vi "determineConfigTabUIPath.vi"(8 "error in (no error)":errorcluster, 11 "ConfigurationTabUI in":refnum<class "ConfigurationTabUI.lvclass">) -> (0 "error out":errorcluster, 2 "cfgTabUIPath":path, 3 "ConfigurationTabUI out":refnum<class "ConfigurationTabUI.lvclass">)   [LabVIEW 2012, in "ExampleConfiguration.lvlib" / "ConfigurationTabUI.lvclass"]
doc: "Determines the path to configTabUI.vi."
uses:
  ConfigurationTabUI.lvclass
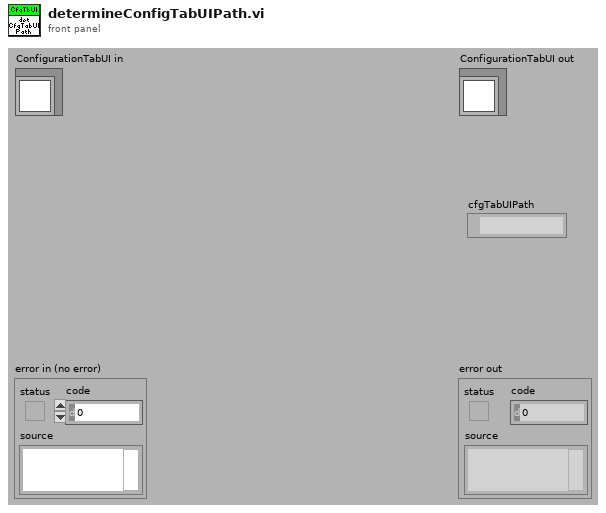
[diagram p1: front panel]
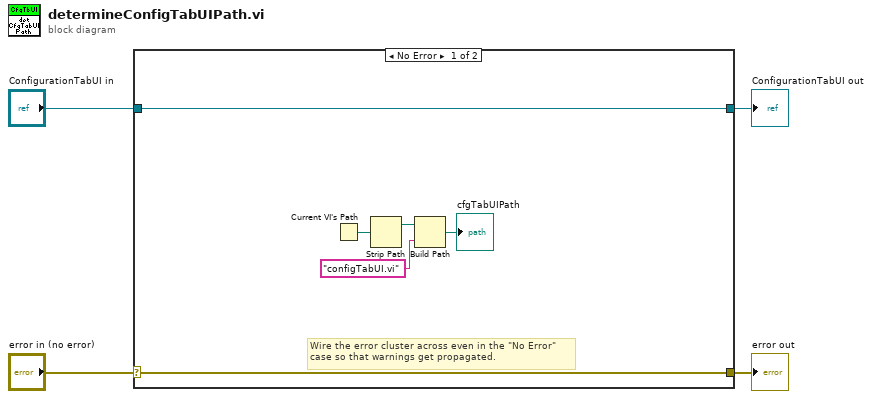
[diagram p0: block diagram]
diagram:
  n1 = case shown="No Error" "error in (no error)" {
    selector: "error in (no error)" -> [w9 w12]
    tunnel: [w9 w12] -> w3
    tunnel: [w10 w11] -> w1
    tunnel: "ConfigurationTabUI in" -> [w10 w11]
    frame No Error {
      # "Wire the error cluster across even in the \"No Error\"\ncase so that warnings get propagated."
      n2 = Current VI's Path() -> (path=w8:path)
      n3 = Strip Path(path=w8) -> (stripped path=w7:path)  [unwired: 1 out]
      n4 = Build Path(base path=w7, name or relative path="configTabUI.vi") -> (appended path=→"cfgTabUIPath":path)
    }
    frame Error {
    }
  }
  "error out" <- w3
  "ConfigurationTabUI out" <- w1
